vi "Serialize as XML.vi"(8 "error in (no error)":errorcluster, 9 "Nesting Level":i32, 11 "Data Item in":refnum<class "Data Item.lvclass">) -> (0 "error out":errorcluster, 2 "XML Fragment":string, 3 "Data Item out":refnum<class "Data Item.lvclass">)   [LabVIEW 2026, in "VILab.lvlib" / "Data Item.lvclass"]
uses:
  Data Item.lvclass
  Data Item.lvclass/Data Item.ctl
  VILab.lvlib
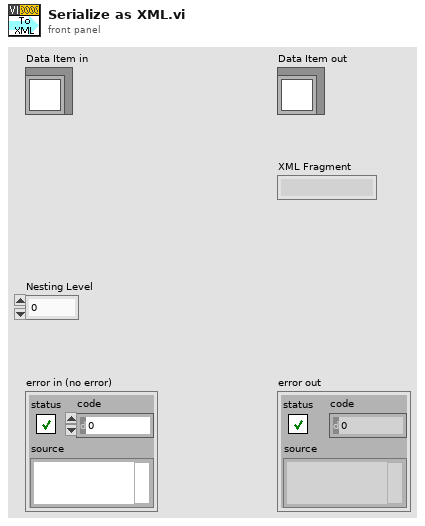
[diagram p1: front panel]
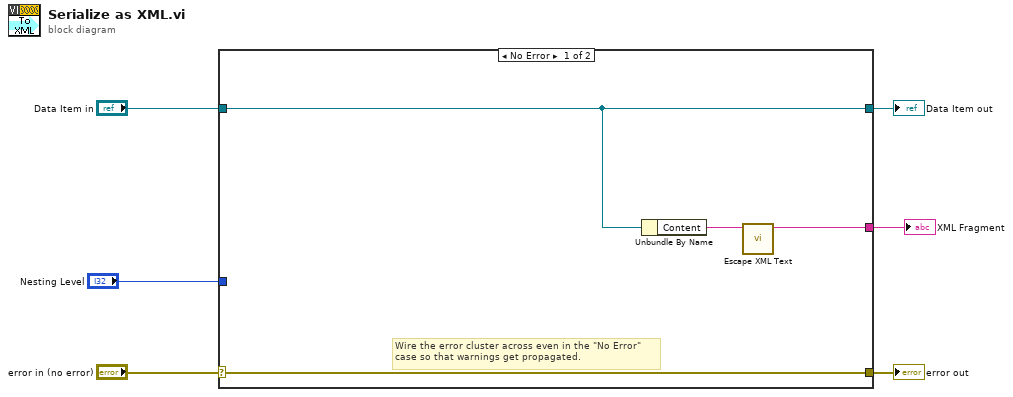
[diagram p0: block diagram]
diagram:
  n1 = case shown="No Error" "error in (no error)" {
    selector: "error in (no error)" -> [w10 w12]
    tunnel: [w10 w12] -> w5
    tunnel: [w9 w11] -> w3
    tunnel: "Data Item in" -> [w9 w11]
    tunnel: [w7 _] -> w2
    tunnel: "Nesting Level" -> [_ _]
    frame No Error {
      # "Wire the error cluster across even in the \"No Error\"\ncase so that warnings get propagated."
      n2 = Unbundle By Name(w9) -> ("Content"=w8:string)
      n3 = call "Escape XML Text.vi"("String"=w8) -> ("Escaped String"=w7:string)  [unwired: 10 in]
    }
    frame Error {
    }
  }
  "error out" <- w5
  "Data Item out" <- w3
  "XML Fragment" <- w2
